vi "Calculate Gain and Offset.vi"(8 "error in":errorcluster, 10 "device sessions":T2, 11 "measurement configuration":T3={"Input channel"=0, "Full scale range"=10.0, "Transition span"=1.5, "Transition step size"=800000.0, "Analog source resource name"="", "Digital capture resource name"="", "Digital capture sample rate"=-1.0, "Digital capture samples"=10000, "DMM resource name"="", "DMM range"=800000.0, "DMM resolution"=5.5} {"DMM range" format="%#_6pV"; "Digital capture sample rate" format="%#_6pS/s"; "Transition step size" format="%#_gLSB"; "Transition span" format="%#_gLSB"; "Full scale range" format="%#_6pV"}) -> (0 "error out":errorcluster, 2 "Offset":dbl, 3 "Gain":dbl)   [LabVIEW 2021, in "Full Scale Error_ADC.lvlib"]
uses:
  Full Scale Error_ADC.lvlib
  Measurement Configuration.ctl
  <vilib>/gRPC/LabVIEW gRPC Library/Shared/grpcId.ctl
  <vilib>/Analysis/1siggen.llb/Ramp Pattern by Samples.vi
  <vilib>/DAQmx/write.llb/DAQmx Write (Analog 1D DBL 1Chan NSamp).vi
  <vilib>/Analysis/baseanly.llb/Mean (DBL).vi
  <vilib>/DAQmx/miscellaneous.llb/DAQmx Fill In Error Info.vi
  <vilib>/Analysis/NI_AALBase.lvlib
  <vilib>/Analysis/NI_AALPro.lvlib
  shared/digitalInterface/client/dcvmDPI_AD7606B_clientImpl/dcvmDPI_AD7606B_clientImpl.lvlib
  <vilib>/gRPC/LabVIEW gRPC Library/grpc-lvsupport-release.lvlib
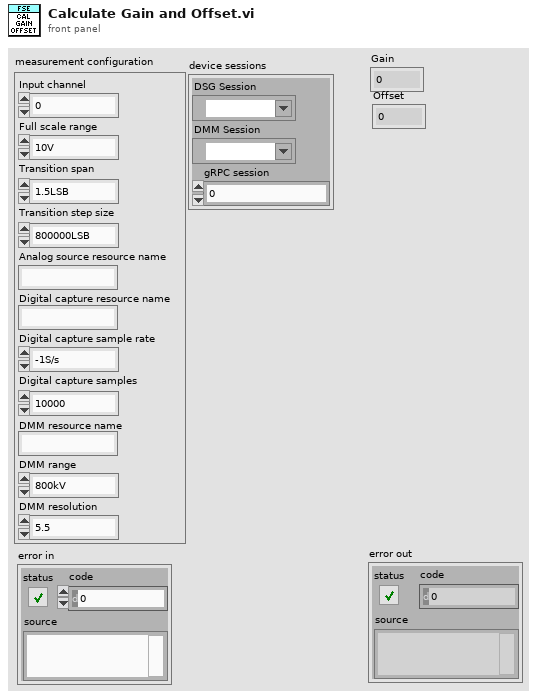
[diagram p1: front panel]
types:
  T1 = typedef "grpc-lvsupport-release.lvlib/grpcId.ctl" = u64
  T2 = cluster{"DSG Session":refnum<k21>, "DMM Session":refnum<k15>, "gRPC session":T1}
  T3 = typedef "Full Scale Error_ADC.lvlib/Measurement Configuration.ctl" = cluster{"Input channel":i32, "Full scale range":dbl, "Transition span":dbl, "Transition step size":dbl, "Analog source resource name":string, "Digital capture resource name":string, "Digital capture sample rate":dbl, "Digital capture samples":u32, "DMM resource name":string, "DMM range":dbl, "DMM resolution":dbl}
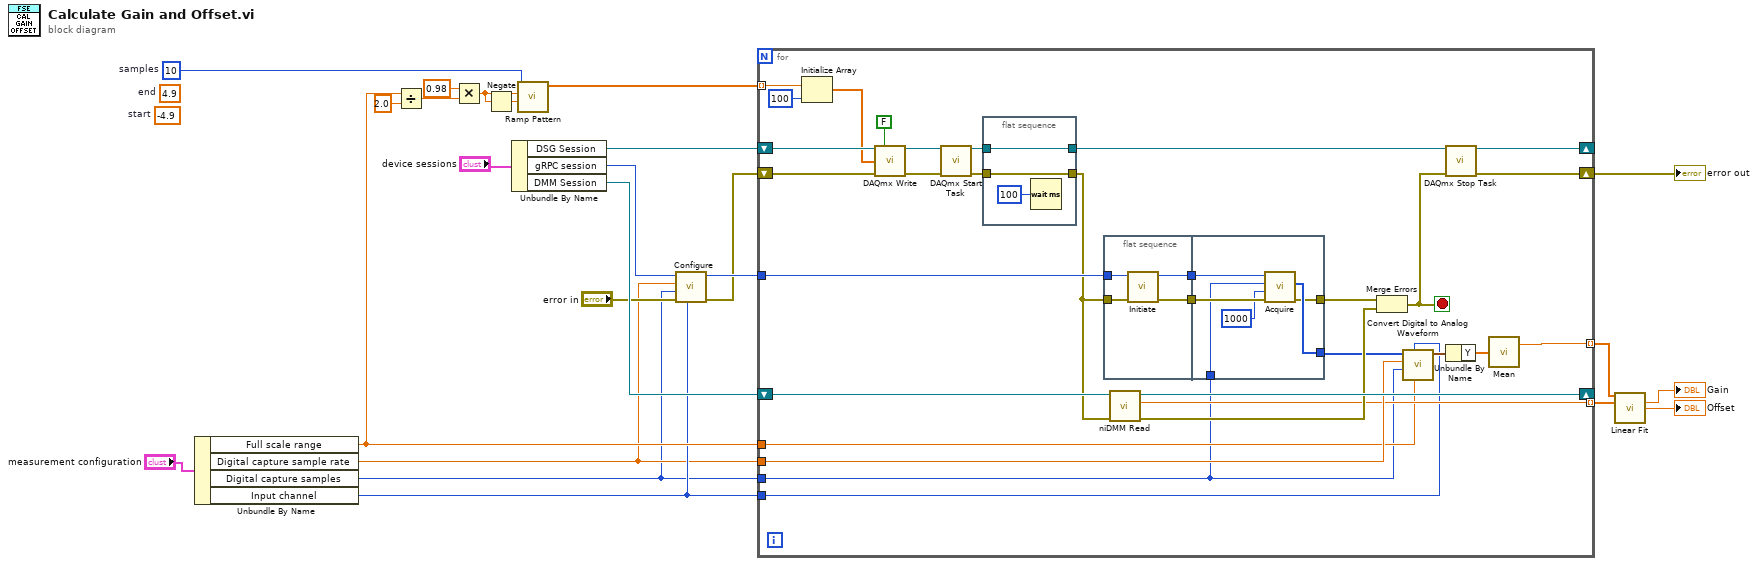
[diagram p0: block diagram]
diagram:
  (unwired) -4.9  # start
  (unwired) 4.9  # end
  w15 = 10  # samples
  n1 = Unbundle By Name("measurement configuration") -> ("Full scale range"=w9:dbl, "Digital capture sample rate"=w3:dbl, "Digital capture samples"=w2:u32, "Input channel"=w5:i32)
  n2 = Divide(x=w9, y=2.0) -> (x/y=w13:dbl)
  n3 = Multiply(x=0.98, y=w13) -> (x*y=w11:dbl)
  n4 = Negate(x=w11) -> (-x=w10:dbl)
  n5 = Unbundle By Name("device sessions") -> ("DSG Session"=w23:refnum<k21>, "gRPC session"=w6:T1, "DMM Session"=w22:refnum<k15>)
  n6 = call-poly <vilib>:"Ramp Pattern.vi"("start"=w10, "end"=w11, "samples"=w15) -> ("Ramp Pattern"=w24:dbl[])  [unwired: 7 in, 1 out]
  n7 = call "Configure.vi"("Input channel"=w5, "error in"="error in", "Digital capture samples"=w2, "Digital capture sample rate"=w3, "gRPC session in"=w6) -> ("error out"=w1:errorcluster, "gRPC session out"=w7:T1)  [unwired: 5 in]
  n8 = for {
    tunnel: w24 -> [w55] mode=indexing
    shift-right: [w41] -> _
    shift-left: w23 -> [w53]
    shift-right: [w45] -> _
    shift-left: w22 -> [w46]
    tunnel: w3 -> [w44]
    tunnel: w2 -> [w27]
    shift-right: [w37] -> w20
    shift-left: w1 -> [w36]
    tunnel: [w35] -> w18 mode=indexing
    tunnel: [w34] -> w19 mode=indexing
    tunnel: w5 -> [w33]
    tunnel: w9 -> [w32]
    tunnel: w7 -> [w31]
    stop <- w39 stop-if-true
    n9 = Initialize Array(w55, 100 ("dimension size")) -> (w47:dbl[])
    n10 = call-poly <vilib>:"DAQmx Write.vi"("task/channels in"=w53, "auto start"=FALSE, "data"=w47, "error in"=w36) -> ("task out"=w51:refnum<k21>, "error out"=w50:errorcluster)  [unwired: 9 in, 1 out]
    n11 = call <vilib>:"DAQmx Start Task.vi"("task/channels in"=w51, "error in"=w50) -> ("task out"=w48:refnum<k21>, "error out"=w49:errorcluster)  [unwired: 12 in]
    n12 = flat-sequence {
      tunnel: w49 -> [w66]
      tunnel: w48 -> [w67]
      tunnel: [w67] -> w40
      tunnel: [w66] -> w30
      frame #0 {
        n13 = Wait (ms)(milliseconds to wait=u32 100) -> ()  [unwired: 1 out]
      }
    }
    n14 = flat-sequence {
      tunnel: w31 -> [w59]
      tunnel: w30 -> [w58]
      tunnel: [w57] -> w29
      tunnel: [w56] -> w28
      tunnel: w29 -> [w65]
      tunnel: w28 -> [w64]
      tunnel: w27 -> [w63]
      tunnel: [w61] -> w26
      tunnel: [w60] -> w25
      frame #0 {
        n15 = call "Initiate.vi"("error in"=w58, "gRPC session in"=w59) -> ("error out"=w56:errorcluster, "gRPC session out"=w57:T1)  [unwired: 8 in]
      }
      frame #1 {
        n16 = call "Acquire.vi"("error in"=w64, "Timeout (ms)"=1000, "Digital capture samples"=w63, "gRPC session in"=w65) -> ("error out"=w60:errorcluster, "Digital waveform"=w61:u32[])  [unwired: 5 in, 1 out]
      }
    }
    n17 = call <instrlib>:"niDMM Read.vi"("error in (no error)"=w30, "instrument handle"=w46) -> ("error out"=w42:errorcluster, "Measurement"=w34:dbl, "instrument handle out"=w45:refnum<k15>)  [unwired: 7 in]
    n18 = Merge Errors(w25, w42) -> (w39:errorcluster)
    n19 = call "Convert Digital to Analog Waveform.vi"("full scale range"=w32, "channel index"=w33, "Number of samples"=w27, "Sample rate"=w44, "Digital waveform in"=w26) -> ("Waveform"=w43:waveform(dbl))  [unwired: 4 in, 2 out]
    n20 = call <vilib>:"DAQmx Stop Task.vi"("task/channels in"=w40, "error in"=w39) -> ("task out"=w41:refnum<k21>, "error out"=w37:errorcluster)  [unwired: 12 in]
    n21 = Unbundle By Name(w43) -> ("Y"=w38:dbl[])
    n22 = call-poly <vilib>:"Mean.vi"("X"=w38) -> ("mean"=w35:dbl)  [unwired: 1 out]
  }
  "error out" <- w20
  n23 = call <vilib>:"Linear Fit.vi"("Y"=w18, "X"=w19) -> ("slope"=→"Gain":dbl, "intercept"=→"Offset":dbl)  [unwired: 9 in, 3 out]
